vi "Init.vi"(8 "Error In":errorcluster, 10 "HAL.lvlib:IConfigure":refnum<class "IConfigure.lvclass">, 11 "object in":refnum<class "Scope PXI.lvclass">) -> (0 "Error Out":errorcluster, 3 "object out":refnum<class "Scope PXI.lvclass">)   [LabVIEW 2023]
uses:
  Interfaces/IConfigure/IConfigure.lvclass
  Scope PXI.lvclass
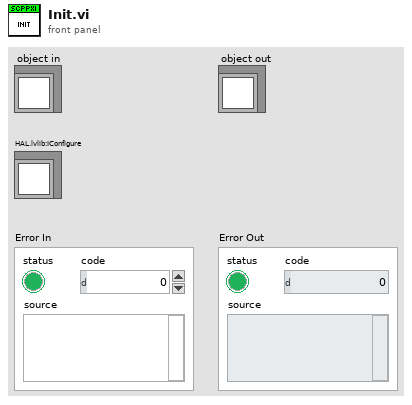
[diagram p1: front panel]
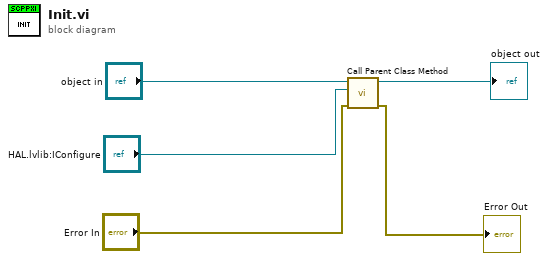
[diagram p0: block diagram]
diagram:
  n1 = call-parent "Call Parent Class Method"("Error In"="Error In", "HAL.lvlib:IConfigure"="HAL.lvlib:IConfigure", "object in"="object in") -> ("Error Out"=→"Error Out":errorcluster, "object out"=→"object out":refnum<class "Scope PXI.lvclass">)  [unwired: 7 in]
